vi "Get AI names from PGserver2.vi"(6 "conn":T2={"host"="localhost", "port"="5432", "client_encoding"="WIN1251", "dbname"="data", "user"="postgres", "password"=""}, 8 "error in (no error)":errorcluster, 9 "AIParamColumns":string[](array[string])=["fcode_full", "fname", "process_units"], 10 "AIParamTable":string="fa_3", 11 "AIParameters":string[](array[string])) -> (0 "error out":errorcluster, 3 "Names table":string[][](array[string]))   [LabVIEW 2019, in "Inputs.lvlib"]
uses:
  Inputs.lvlib
  Database/ctl/Coninfo.ctl
  Database/PostgreSQL2LabVIEW/libpqlv/src/PQfinish.vi
  Database/PostgreSQL2LabVIEW/libpqlv/src/PQconnectdb.vi
  Database/PostgreSQL2LabVIEW/libpqlv/src/PQerrorMessage.vi
  Database/PostgreSQL2LabVIEW/libpqlv/src/PQstatus.vi
  <vilib>/dlg_ctls.llb/Space Constant.vi
  Database/Progress.vi
  Database/PostgreSQL.lvlib
  Database/PostgreSQL2LabVIEW/libpqUtility/libpqutility.lvlib
  Database/PostgreSQL2LabVIEW/libpqUtility64/libpqutility64.lvlib
panel:
  out "PQStatus":T1(ring)
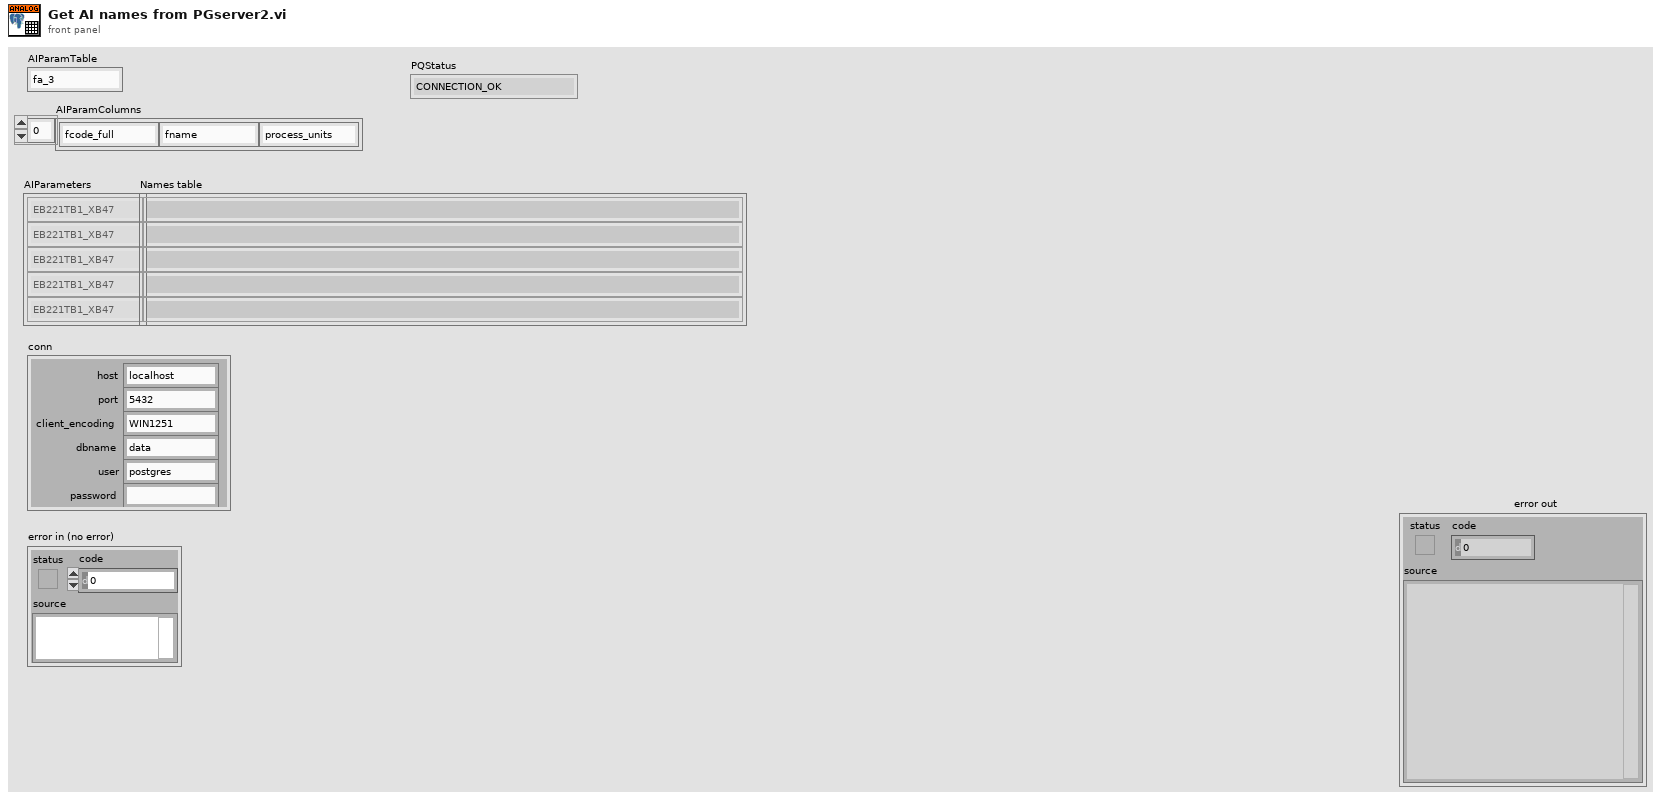
[diagram p1: front panel]
types:
  T1 = enum32{"CONNECTION_OK", "CONNECTION_BAD", "CONNECTION_STARTED", "CONNECTION_MADE", "CONNECTION_AWAITING_RESPONSE", "CONNECTION_AUTH_OK", "CONNECTION_SETENV", "CONNECTION_SSL_STARTUP", "CONNECTION_NEEDED"}
  T2 = typedef "PostgreSQL.lvlib/Coninfo.ctl" = cluster{"host":string, "port":string, "client_encoding":string, "dbname":string, "user":string, "password":string}
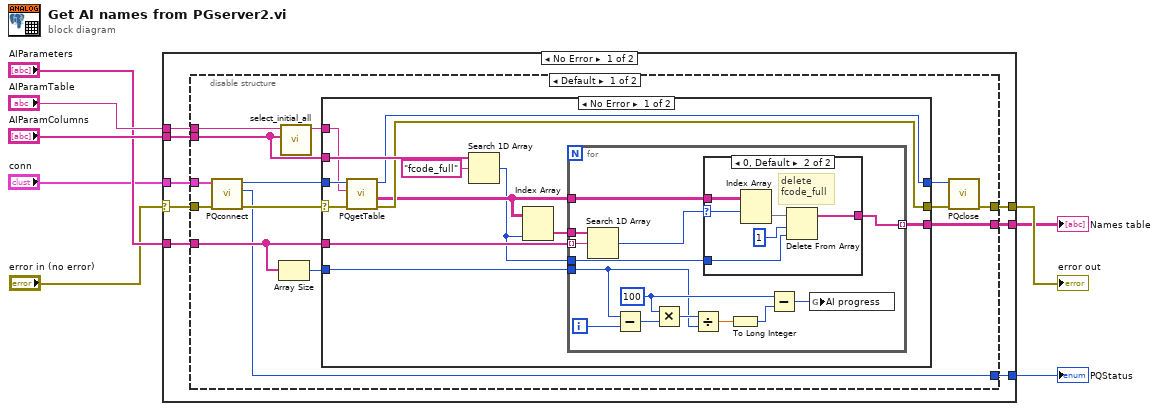
[diagram p0: block diagram]
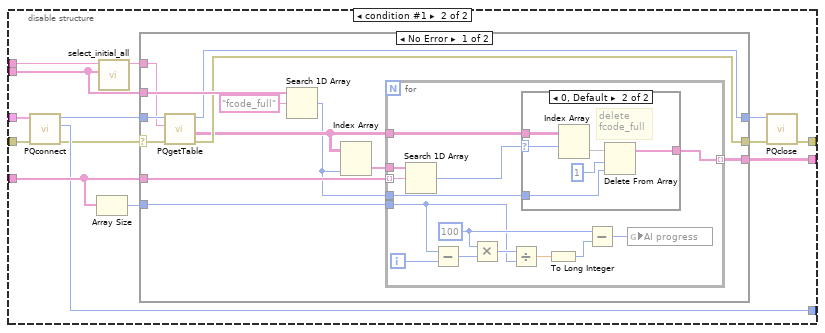
[diagram p4: hidden frame]
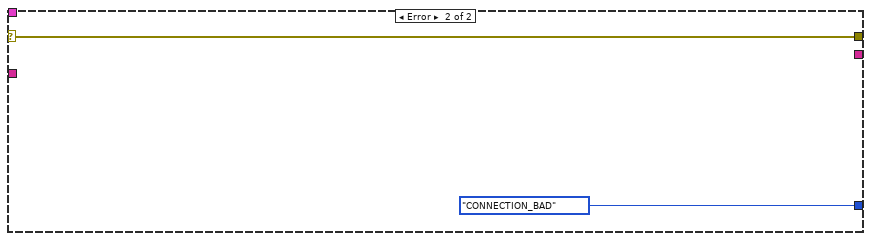
[diagram p7: hidden frame]
diagram:
  n1 = case shown="No Error" "error in (no error)" {
    selector: "error in (no error)" -> [w13 w116]
    tunnel: [w9 w116] -> w8
    tunnel: [w10 _] -> w7
    tunnel: "AIParamColumns" -> [w16 _]
    tunnel: "conn" -> [w12 _]
    tunnel: "AIParamTable" -> [w15 _]
    tunnel: "AIParameters" -> [w14 _]
    tunnel: [w11 T1."CONNECTION_BAD" ("PQStatus")] -> w1
    frame No Error {
      n2 = disable-structure shown="Default" {
        disable-tunnel: w16 -> [w19 w77]
        disable-tunnel: w15 -> [w21 w76]
        disable-tunnel: w14 -> [w25 w75]
        disable-tunnel: w13 -> [w23 w69]
        disable-tunnel: w12 -> [w24 w70]
        disable-tunnel: [w22 w67] -> w11
        disable-tunnel: [w18 w74] -> w10
        disable-tunnel: [w17 w71] -> w9
        frame condition #0 (active) {
          n3 = call "PQconnect.vi"("error in (no error)"=w23, "conninfo"=w24) -> ("error out"=w28:errorcluster, "PQStatus"=w22:T1, "conn"=w29:u32)  [unwired: 7 in]
          n4 = Array Size(array=w25) -> (size(s)=w30:i32)
          n5 = call "select_initial_all.vi"("Column table"=w19, "table"=w21) -> ("parameters"=w20:string)  [unwired: 8 in, 1 out]
          n6 = case shown="No Error" w28 {
            selector: w28 -> [w39 w64]
            tunnel: w25 -> [w43 _]
            tunnel: w30 -> [w42 _]
            tunnel: w20 -> [w33 _]
            tunnel: [w34 w64] -> w26
            tunnel: [w35 w65] -> w27
            tunnel: [w41 _] -> w18
            tunnel: w29 -> [w40 w65]
            tunnel: w19 -> [w36 _]
            frame No Error {
              n7 = call "PQgetTable.vi"("error in"=w39, "query"=w33, "conn"=w40) -> ("error out"=w34:errorcluster, "Data"=w32:string[][], "conn_out"=w35:u32)  [unwired: 4 in, 2 out]
              n8 = Search 1D Array(1D array=w36, element="fcode_full" ("table")) -> (index of element=w31:i32)  [unwired: 1 in]
              n9 = Index Array(array=w32, index (col)=w31) -> (element=w37:string[])  [unwired: 1 in]
              n10 = for {
                tunnel: w42 -> [w50]
                tunnel: w43 -> [w47] mode=indexing
                tunnel: [w49] -> w41 mode=indexing
                tunnel: w37 -> [w48]
                tunnel: w32 -> [w45]
                tunnel: w31 -> [w44]
                i -> [w51]
                w55 = 100 ("y")
                n11 = Search 1D Array(1D array=w48, element=w47) -> (index of element=w46:i32)  [unwired: 1 in]
                n12 = Subtract(x=w50, y=w51) -> (x-y=w54:i32)
                n13 = Multiply(x=w55, y=w54) -> (x*y=w57:i32)
                n14 = Divide(x=w57, y=w50) -> (x/y=w53:dbl)
                n15 = case shown="0, Default" w46 {
                  selector: w46 -> [_ w62]
                  tunnel: w45 -> [_ w63]
                  tunnel: [_ w61] -> w49
                  tunnel: w44 -> [_ w59]
                  frame -1 {
                  }
                  frame 0, Default {
                    # "delete\nfcode_full"
                    n16 = Index Array(array=w63, index (row)=w62) -> (element=w60:string[])  [unwired: 1 in]
                    n17 = Delete From Array(array=w60, length=1, index=w59) -> (array with subset deleted=w61:string[])  [unwired: 1 out]
                  }
                }
                n18 = To Long Integer(number=w53) -> (32bit integer=w52:i32)
                n19 = Subtract(x=w55, y=w52) -> (x-y=w56:i32)
                n20 = global write "Progress.vi" "AI progress"(w56) -> ()
              }
            }
            frame Error {
            }
          }
          n21 = call "PQclose.vi"("error in (no error)"=w26, "conn"=w27) -> ("error out"=w17:errorcluster)  [unwired: 9 in]
        }
        frame condition #1 {
          n22 = call "PQconnect.vi"("error in (no error)"=w69, "conninfo"=w70) -> ("error out"=w66:errorcluster, "PQStatus"=w67:T1, "conn"=w68:u64)  [unwired: 7 in]
          n23 = Array Size(array=w75) -> (size(s)=w79:i32)
          n24 = call "select_initial_all.vi"("Column table"=w77, "table"=w76) -> ("parameters"=w78:string)  [unwired: 8 in, 1 out]
          n25 = case shown="No Error" w66 {
            selector: w66 -> [w84 w113]
            tunnel: w75 -> [w92 _]
            tunnel: w79 -> [w91 _]
            tunnel: w78 -> [w83 _]
            tunnel: [w85 w113] -> w72
            tunnel: [w82 w114] -> w73
            tunnel: [w90 _] -> w74
            tunnel: w68 -> [w86 w114]
            tunnel: w77 -> [w87 _]
            frame No Error {
              n26 = call "PQgetTable.vi"("error in"=w84, "query"=w83, "conn"=w86) -> ("error out"=w85:errorcluster, "Data"=w81:string[][], "conn_out"=w82:u64)  [unwired: 4 in, 2 out]
              n27 = Search 1D Array(1D array=w87, element="fcode_full" ("table")) -> (index of element=w80:i32)  [unwired: 1 in]
              n28 = Index Array(array=w81, index (col)=w80) -> (element=w88:string[])  [unwired: 1 in]
              n29 = for {
                tunnel: w91 -> [w99]
                tunnel: w92 -> [w97] mode=indexing
                tunnel: [w94] -> w90 mode=indexing
                tunnel: w88 -> [w98]
                tunnel: w81 -> [w96]
                tunnel: w80 -> [w93]
                i -> [w100]
                w104 = 100 ("y")
                n30 = Search 1D Array(1D array=w98, element=w97) -> (index of element=w95:i32)  [unwired: 1 in]
                n31 = Subtract(x=w99, y=w100) -> (x-y=w103:i32)
                n32 = Multiply(x=w104, y=w103) -> (x*y=w106:i32)
                n33 = Divide(x=w106, y=w99) -> (x/y=w102:dbl)
                n34 = case shown="0, Default" w95 {
                  selector: w95 -> [_ w111]
                  tunnel: w96 -> [_ w112]
                  tunnel: [_ w110] -> w94
                  tunnel: w93 -> [_ w108]
                  frame -1 {
                  }
                  frame 0, Default {
                    # "delete\nfcode_full"
                    n35 = Index Array(array=w112, index (row)=w111) -> (element=w109:string[])  [unwired: 1 in]
                    n36 = Delete From Array(array=w109, length=1, index=w108) -> (array with subset deleted=w110:string[])  [unwired: 1 out]
                  }
                }
                n37 = To Long Integer(number=w102) -> (32bit integer=w101:i32)
                n38 = Subtract(x=w104, y=w101) -> (x-y=w105:i32)
                n39 = global write "Progress.vi" "AI progress"(w105) -> ()
              }
            }
            frame Error {
            }
          }
          n40 = call "PQclose.vi"("error in (no error)"=w72, "conn"=w73) -> ("error out"=w71:errorcluster)  [unwired: 9 in]
        }
      }
    }
    frame Error {
    }
  }
  "error out" <- w8
  "Names table" <- w7
  "PQStatus" <- w1
